vi "DIO_Query.vi"(0 "System no.":i32=1 min=1 max=4 step=1, 2 "DI's to query":string[](array[string]), 3 "All DI's?":bool, 4 "DI identifier?":bool=TRUE, 5 "error in":errorcluster, 6 "Invert order for TVI?":bool=TRUE) -> (14 "DI value":bool[](array[boolean]), 19 "error out":errorcluster)   [LabVIEW 2020]
doc: "Returns digital input values for queried digital inputs. Uses TIO?.vi (GCS 1.0 and 2.0) and TVI?.vi (GCS 1.0) to determine available DI identifiers if All DI's = TRUE and DI identifier = TRUE. If Query pattern? = TRUE, returns binary pattern for the digital input status of all channels.\n\nC-413: If All DI's = TRUE, then DI identifier must be FALSE. Invert order for TVI? is not valid. DI's to query are 1 to . Query pattern? is not valid.\n\nC-702, C-848, C-880: If All DI's = TRUE, then DI identifier can be FALSE and Invert order for TVI? must be TRUE. Query pattern? is not valid.\n\nC-843, C-843.PM, C-865, C-866: If All DI's = TRUE, then DI identifier must be TRUE and Invert order for TVI? must be FALSE. Query pattern? is not valid..\n\nC-867, C-884, E-861, E-871, E-873, E-874, Mercury_GCS: If All DI's = TRUE, then DI identifier must be FALSE. Invert order for TVI? is not valid. DI's to query are 1-4. Query pattern? can be TRUE.\n\nC-877: If All DI's = TRUE, then DI identifier must be FALSE. Invert order for TVI? is not valid. DI's to query are 1-4. Query pattern? can be TRUE.Check HLP?/HELP answer to find out if DIO is supported\n\nC-891: If All DI's = TRUE, then DI identifier must be FALSE. Invert order for TVI? is not valid. . If All DI's = FALSE, only one DI to query per command allowed and DI's to query can be 1 to 4. Query pattern? can be TRUE.\n\nE-517, E-518: If All DI's = TRUE, then DI identifier can be FALSE. Invert order for TVI? is not valid. DI's to query are 1-3. Query pattern? is not valid.\n\nE-709, E-727: If All DI's = TRUE, then DI identifier can be FALSE. Invert order for TVI? is not valid. Query pattern? is not valid. \n\nE-754: If All DI's = TRUE, then DI identifier can be FALSE. Invert order for TVI? is not valid. DI's to query are 1-2. Query pattern? is not valid.\n\nE-761: All DI's = FALSE. DI's to query are \"1\". Query pattern? is not valid. Note that the E-761 has no genuine digital input lines, but the analog input is internally interpreted as digital input for triggering tasks (see E-761 user manual), and its signal state can be queried by this command. If the voltage on the analog input is < 0.8 V, the signal is interpreted as LOW, if the voltage is = 2.4 V, the signal is interpreted as HIGH.\n\nC-887, F-206, M-8X0: If All DI's = TRUE, then DI identifier must be FALSE. Invert order for TVI? is not valid. DI's to query are 1 to 8. Query pattern? can be TRUE. Only for GCS syntax version = GCS 2.0 or higher (Check with CSV?.vi. If CSV?.vi is not supported, syntax version is GCS 1.0).\n\nE-872: If All DI's = TRUE, then DI identifier must be FALSE. Invert order for TVI? is not valid. DI's can be queried with TIO?.vi. Query pattern? can be TRUE.\n\nHydra: If All DI's = TRUE, then DI identifier must be FALSE. Invert order for TVI? is not valid. DI's to query are 1-2. Query pattern? can be TRUE.\n\nMercury: All DI's must be FALSE. DI's to query can be A-D, E-H, I-L etc., see GCS DLL Manual for details. Query pattern? is not valid."
panel:
  out "DI pattern":u32 format="%x"
  in  "Query pattern?":bool
  # "Returns digital input values for queried digital inputs. Uses \"TIO?.vi\" (GCS I and\nII) and \"TVI?.vi\" (GCS I) to determine available DI identifiers if \"All DI's\" = TRUE\nand DI identifier = TRUE."
  # "Query"
  # "If all DI's:"
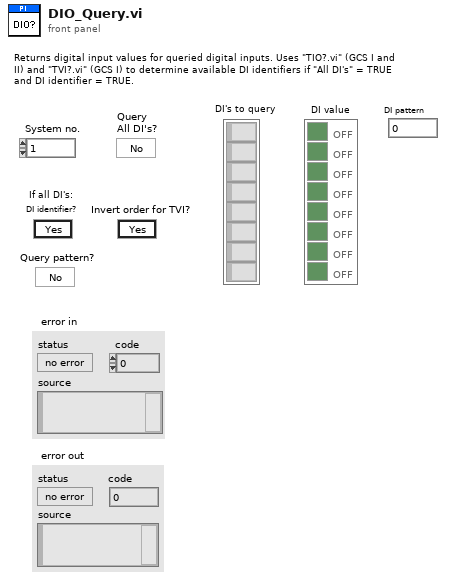
[diagram p1: front panel]
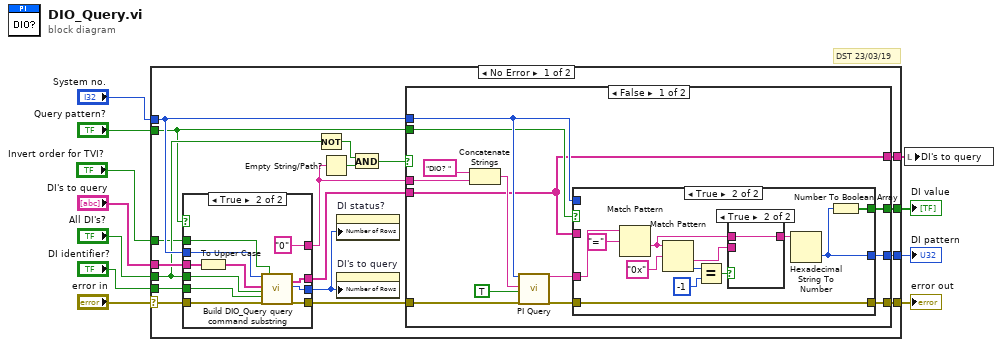
[diagram p0: block diagram]
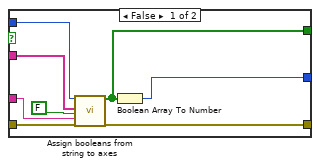
[diagram p2: hidden frame]
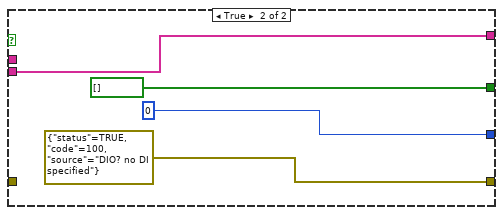
[diagram p4: hidden frame]
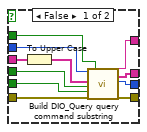
[diagram p5: hidden frame]
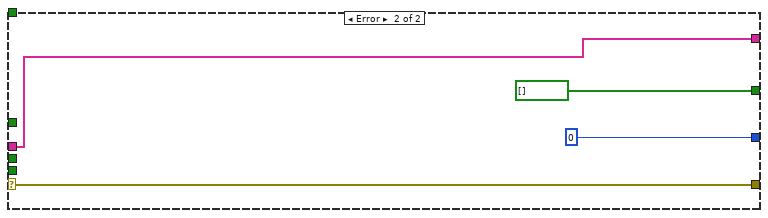
[diagram p6: hidden frame]
diagram:
  # "DST 23/03/19"
  n1 = case shown="No Error" "error in" {
    selector: "error in" -> [w17 w92]
    tunnel: [w19 bool[] [] ("Booleans")] -> w11
    tunnel: "DI's to query" -> [w29 w91]
    tunnel: [w28 w92] -> w9
    tunnel: "DI identifier?" -> [w27 _]
    tunnel: "System no." -> [w26 _]
    tunnel: "All DI's?" -> [w22 _]
    tunnel: "Invert order for TVI?" -> [w21 _]
    tunnel: [w20 u32 0] -> w4
    tunnel: "Query pattern?" -> [w18 _]
    tunnel: [w13 w91] -> w1
    frame No Error {
      n2 = case shown="True" w18 {
        tunnel: w29 -> [w79 w90]
        tunnel: w27 -> [w77 w88]
        tunnel: [w76 "0" ("Command substring")] -> w16
        tunnel: w26 -> [w75 w87]
        tunnel: [w74 w86] -> w24
        tunnel: w17 -> [w73 w85]
        tunnel: [w72 w84] -> w23
        tunnel: w22 -> [w71 w83]
        tunnel: w21 -> [w70 w82]
        tunnel: [w69 w81] -> w14
        frame False {
          n3 = To Upper Case(1:w79) -> (0:w78:string[])
          n4 = call "Build DIO_Query query command substring.vi"("System no."=w75, "DI's to query in"=w78, "Query all DI's?"=w71, "For all DI's: use\nDI identifier?"=w77, "error in"=w73, "For all DI's: \nInvert order for TVI?"=w70) -> ("Command substring"=w76:string, "DI's to query out"=w69:string[], "Number of rows"=w74:u32, "error out"=w72:errorcluster)  [unwired: 10 out]
        }
        frame True {
          n5 = To Upper Case(1:w90) -> (0:w89:string[])
          n6 = call "Build DIO_Query query command substring.vi"("System no."=w87, "DI's to query in"=w89, "Query all DI's?"=w83, "For all DI's: use\nDI identifier?"=w88, "error in"=w85, "For all DI's: \nInvert order for TVI?"=w82) -> ("DI's to query out"=w81:string[], "Number of rows"=w86:u32, "error out"=w84:errorcluster)  [unwired: 11 out]
        }
      }
      n7 = Not(x=w22) -> (.not. x?=w25:bool)
      n8 = Empty String/Path?(string/path=w16) -> (empty?=w15:bool)
      n9 = property on="DI status?" class="Arr (strict)"("Number of Rows"=w24) -> ()  [unwired: 2 in, 2 out]
      n10 = property on="DI's to query" class="Arr (strict)"("Number of Rows"=w24) -> ()  [unwired: 2 in, 2 out]
      n11 = And(x=w25, y=w15) -> (x .and. y?=w12:bool)
      n12 = case shown="False" w12 {
        tunnel: [w38 errorcluster {"status"=TRUE, "code"=100, "source"="DIO? no DI specified"} ("error out")] -> w28
        tunnel: w26 -> [w39 _]
        tunnel: w23 -> [w37 _]
        tunnel: [w36 u32 0] -> w20
        tunnel: [w35 bool[] [] ("Boolean array")] -> w19
        tunnel: w18 -> [w34 _]
        tunnel: w16 -> [w31 _]
        tunnel: w14 -> [w30 w65]
        tunnel: [w30 w65] -> w13
        frame False {
          n13 = Concatenate Strings("DIO? ", w31) -> (w40:string)
          n14 = call "PI Query.vi"("System no."=w39, "String to send"=w40, "Attach termination char.?"=TRUE ("Attach Linefeed?"), "error in"=w37) -> ("String read"=w33:string, "error out"=w32:errorcluster)  [unwired: 3 in, 11 out]
          n15 = case shown="True" w34 {
            tunnel: w39 -> [w50 _]
            tunnel: w30 -> [w49 _]
            tunnel: w33 -> [w48 w62]
            tunnel: [w47 w58] -> w38
            tunnel: w32 -> [w46 w58]
            tunnel: [w44 w59] -> w36
            tunnel: [w43 w60] -> w35
            frame False {
              n16 = call "Assign booleans from string to axes.vi"("System no."=w50, "Queried axes"=w49, "All axes queried?"=FALSE, "Input String"=w48, "error in"=w46) -> ("Booleans"=w43:bool[], "error out"=w47:errorcluster)  [unwired: 13 out]
              n17 = Boolean Array To Number(Boolean array=w43) -> (number=w44:u32)
            }
            frame True {
              n18 = Match Pattern(string=w62, regular expression="=") -> (after substring=w52:string)  [unwired: 4 out]
              n19 = Match Pattern(string=w52, regular expression="0x") -> (after substring=w57:string, offset past match=w54:i32)  [unwired: 3 out]
              n20 = Equal?(x=w54, y=-1) -> (x = y?=w56:bool)
              n21 = case shown="True" w56 {
                tunnel: w52 -> [_ w64]
                tunnel: [w63 w64] -> w51
                tunnel: w57 -> [w63 _]
                frame False {
                }
                frame True {
                }
              }
              n22 = Hexadecimal String To Number(string=w51) -> (number=w59:u32)  [unwired: 3 out]
              n23 = Number To Boolean Array(number=w59) -> (Boolean array=w60:bool[])
            }
          }
        }
        frame True {
        }
      }
    }
    frame Error {
    }
  }
  "error out" <- w9
  "DI value" <- w11
  "DI pattern" <- w4
  n24 = local write "DI's to query"(w1) -> ()
